vi "Result View.vi"(9 "TestCase map":map{string, map{string, path}}(c390), 10 "Test Tree":refnum<class "Test Tree.lvclass">) -> ()   [LabVIEW 2020]
uses:
  Helper Classes/Test Tree/Test Tree.lvclass
  Helper Classes/Test Tree/Test Tree.lvclass/Test Tree.ctl
panel:
  in  "Test Results":string[](tree)
  in  "Filter fails":bool
  out "Description":string
  out "error out":errorcluster
  in  "error in (no error)":errorcluster
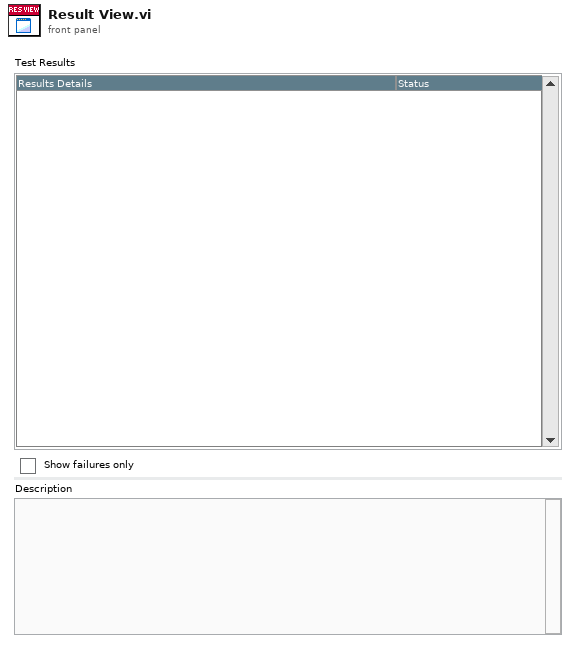
[diagram p1: front panel]
types:
  T1 = cluster{"Message":string, "Message Data":variant}
  T2 = enum32{"Invalid", "Standard", "Closed", "Hidden", "Minimized", "Maximized"}
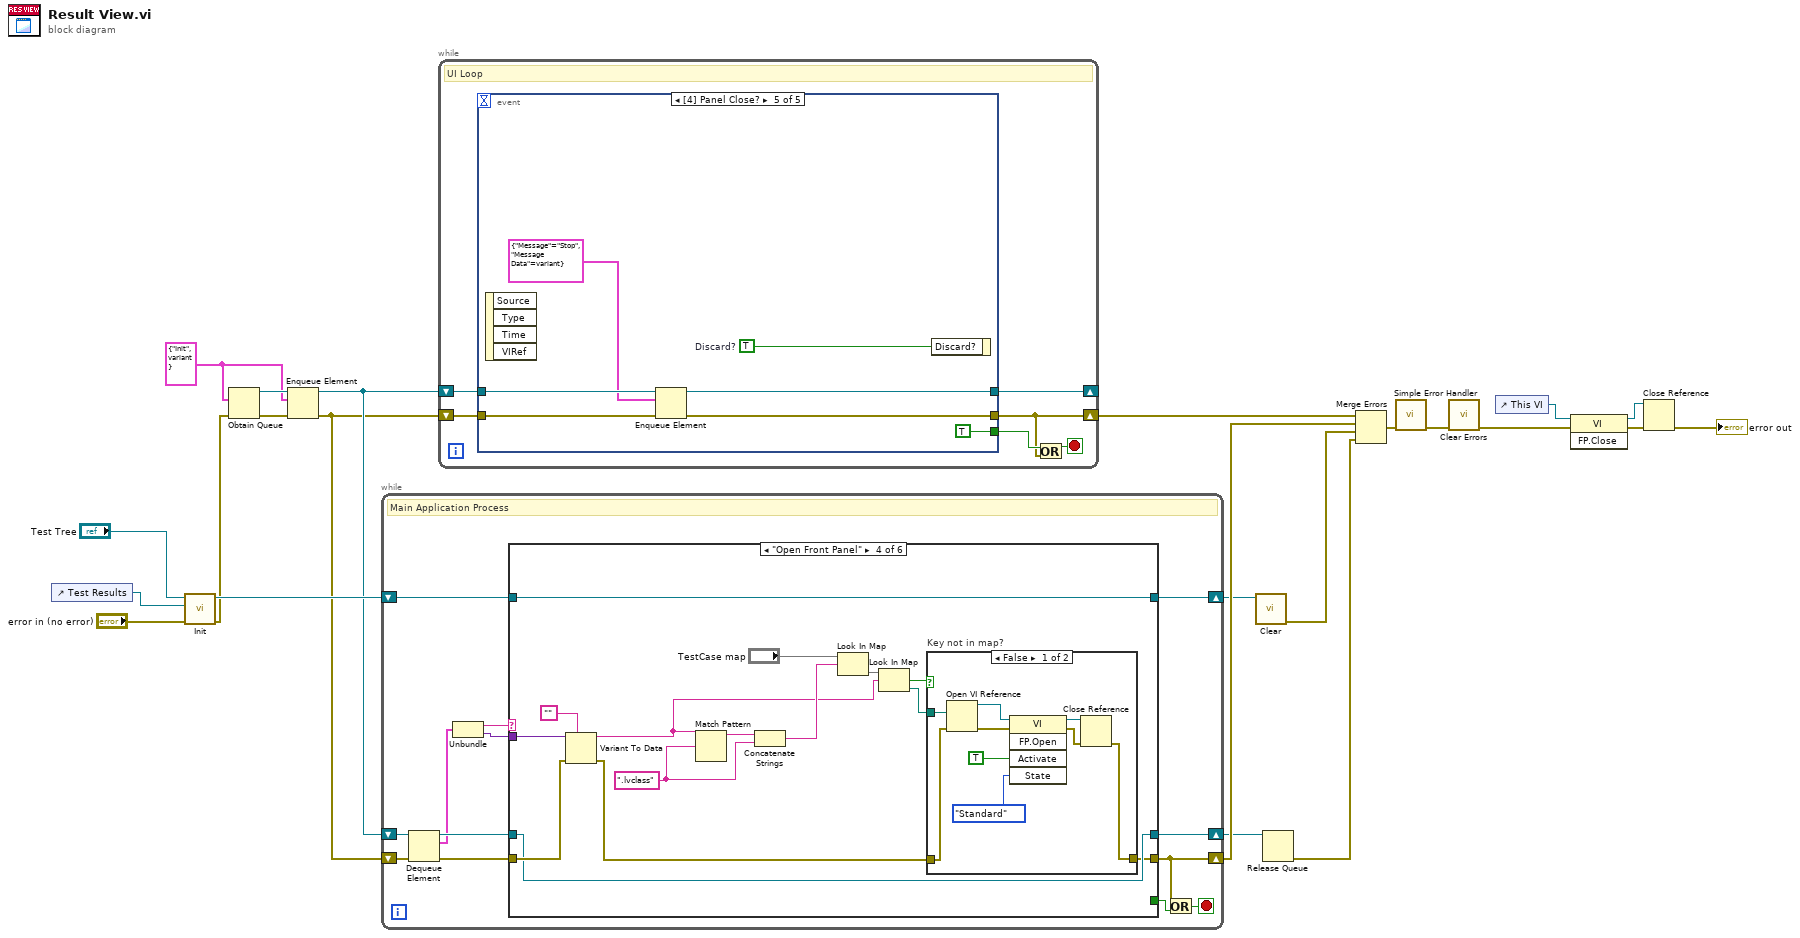
[diagram p0: block diagram]
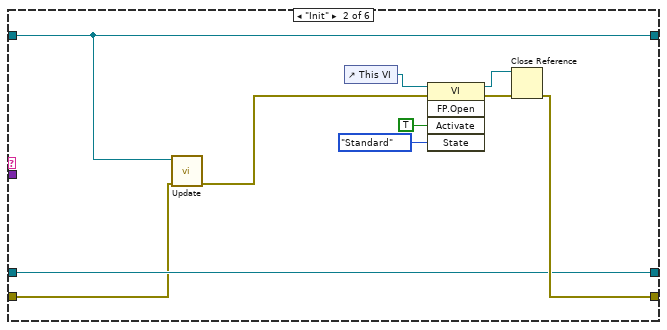
[diagram p3: hidden frame]
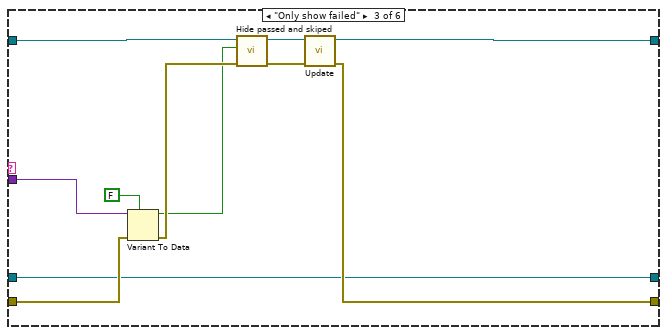
[diagram p4: hidden frame]
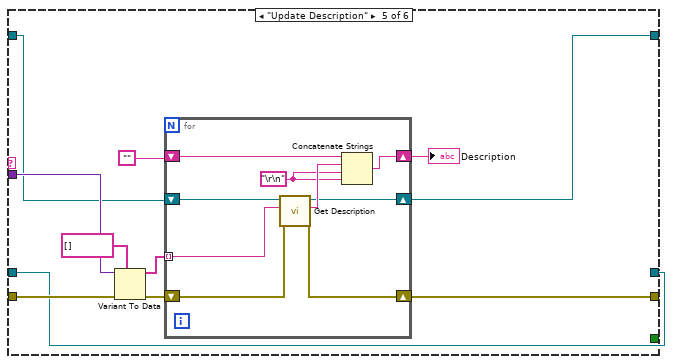
[diagram p6: hidden frame]
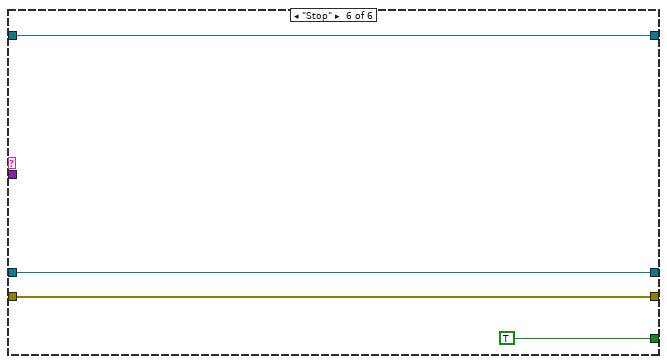
[diagram p7: hidden frame]
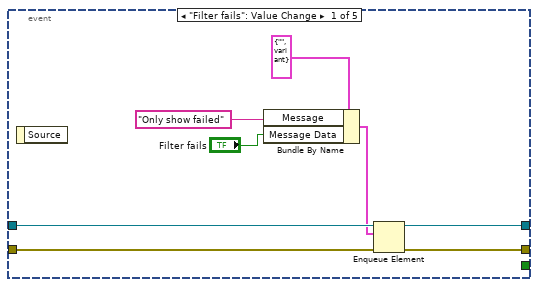
[diagram p8: hidden frame]
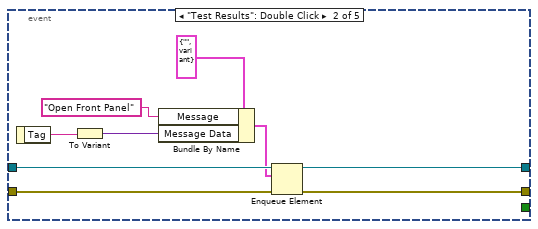
[diagram p9: hidden frame]
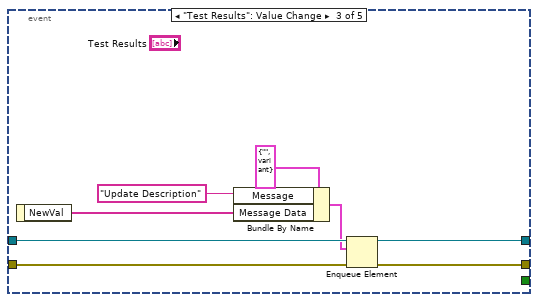
[diagram p10: hidden frame]
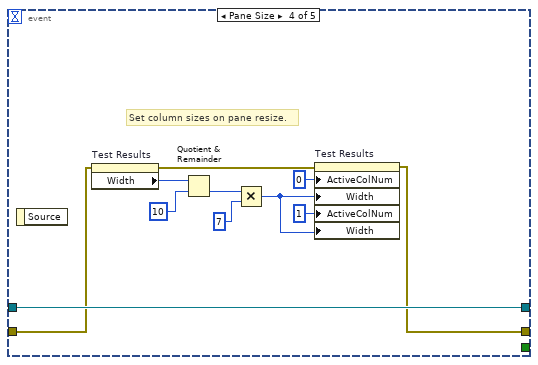
[diagram p11: hidden frame]
diagram:
  w1 = T1 {"Message"="Init", "Message Data"=variant} ("element")
  n1 = control-ref of="Test Results"() -> (w20:refnum<vi>)
  n2 = call-dynamic "Init.vi"("error in (no error)"="error in (no error)", "Test Tree reference"=w20, "Test Tree In"="Test Tree") -> ("error out"=w15:errorcluster, "Test Tree Out"=w16:refnum<class "Test Tree.lvclass">)  [unwired: 7 in]
  n3 = Obtain Queue(element data type=w1, error in (no error)=w15) -> (queue out=w17:refnum<queue>, error out=w13:errorcluster)  [unwired: 3 in, 1 out]
  n4 = Enqueue Element(queue=w17, element=w1, error in (no error)=w13) -> (queue out=w14:refnum<queue>, error out=w12:errorcluster)  [unwired: 1 in, 1 out]
  n5 = while {
    shift-right: [w24] -> w23
    shift-left: w12 -> [w35]
    shift-right: [w31] -> w7
    shift-left: w14 -> [w36]
    shift-right: [w26] -> w8
    shift-left: w16 -> [w27]
    stop <- w25 stop-if-true
    # "Main Application Process"
    n6 = Dequeue Element(queue=w36, error in (no error)=w35) -> (queue out=w34:refnum<queue>, element=w30:T1, error out=w33:errorcluster)  [unwired: 1 in, 1 out]
    n7 = Unbundle(w30) -> ("Message"=w29:string, "Message Data"=w28:variant)
    n8 = case shown="\"Open Front Panel\"" w29 {
      tunnel: w34 -> [w38 w43 w52 w72 w88 w106]
      tunnel: [w38 w43 w52 w72 w88 w106] -> w31
      tunnel: w33 -> [w39 w41 w60 w75 w96 w107]
      tunnel: [w39 w44 w54 w71 w91 w107] -> w24
      tunnel: [_ _ _ _ _ TRUE] -> w32
      tunnel: w28 -> [_ _ w59 w74 w95 _]
      tunnel: w27 -> [w37 w40 w51 w70 w86 w109]
      tunnel: [w37 w40 w50 w70 w87 w109] -> w26
      frame Default {
      }
      frame "Init" {
        n9 = call "Update.vi"("error in (no error)"=w41, "Test Tree In"=w40) -> ("error out"=w42:errorcluster)  [unwired: 8 in, 1 out]
        n10 = control-ref of="This VI"() -> (w47:refnum<vi>)
        n11 = invoke on="Invoke Node" class="VI" method="FP.Open"(reference=w47, error in=w42, "Activate"=TRUE ("Activate?"), "State"=T2."Standard") -> (reference out=w45:refnum<vi>, error out=w46:errorcluster)  [unwired: 1 in, 3 out]
        n12 = Close Reference(reference=w45, error in (no error)=w46) -> (error out=w44:errorcluster)
      }
      frame "Only show failed" {
        n13 = Variant To Data(error in=w60, type=FALSE, Variant=w59) -> (data=w53:bool, error out=w56:errorcluster)
        n14 = call "Hide passed and skiped.vi"("error in (no error)"=w56, "Hide passed/skiped?"=w53, "Test Tree In"=w51) -> ("error out"=w55:errorcluster, "Test Tree Out"=w57:refnum<class "Test Tree.lvclass">)  [unwired: 7 in]
        n15 = call "Update.vi"("error in (no error)"=w55, "Test Tree In"=w57) -> ("error out"=w54:errorcluster, "Test Tree Out"=w50:refnum<class "Test Tree.lvclass">)  [unwired: 8 in]
      }
      frame "Open Front Panel" {
        w64 = ".lvclass" ("regular expression")
        n16 = Variant To Data(error in=w75, type="" ("Empty String Constant"), Variant=w74) -> (data=w63:string, error out=w62:errorcluster)
        n17 = Match Pattern(string=w63, regular expression=w64) -> (before substring=w65:string)  [unwired: 1 in, 3 out]
        n18 = Concatenate Strings(w65, w64) -> (w68:string)
        n19 = Look In Map(map="TestCase map", key=w68) -> (value=w66:map{string, path})  [unwired: 1 in, 1 out]
        n20 = Look In Map(map=w66, key=w63) -> (key not found?=w61:bool, value=w67:path)  [unwired: 1 in]
        n21 = case "Key not in map?" shown="False" w61 {
          tunnel: [w80 w85] -> w71
          tunnel: w67 -> [w79 _]
          tunnel: w62 -> [w76 w85]
          frame False {
            n22 = Open VI Reference(vi path=w79, error in (no error)=w76) -> (vi reference=w78:refnum<vi>, error out=w77:errorcluster)  [unwired: 4 in]
            n23 = invoke class="VI" method="FP.Open"(reference=w78, error in=w77, "Activate"=TRUE ("Activate?"), "State"=T2."Standard") -> (reference out=w81:refnum<vi>, error out=w82:errorcluster)  [unwired: 1 in, 3 out]
            n24 = Close Reference(reference=w81, error in (no error)=w82) -> (error out=w80:errorcluster)
          }
          frame True {
          }
        }
      }
      frame "Update Description" {
        n25 = Variant To Data(error in=w96, type=string[] [], Variant=w95) -> (data=w93:string[], error out=w92:errorcluster)
        n26 = for {
          tunnel: w93 -> [w105] mode=indexing
          shift-right: [w103] -> w91
          shift-left: w92 -> [w104]
          shift-right: [w102] -> w89
          shift-left: "" ("Empty String Constant") -> [w101]
          shift-right: [w97] -> w87
          shift-left: w86 -> [w98]
          w99 = "\r\n" ("End of Line Constant")
          n27 = call "Get Description.vi"("error in (no error)"=w104, "Tag"=w105, "Test Tree In"=w98) -> ("error out"=w103:errorcluster, "Description"=w100:string, "Test Tree Out"=w97:refnum<class "Test Tree.lvclass">)  [unwired: 5 in, 1 out]
          n28 = Concatenate Strings(w101, w100, w99, w99) -> (w102:string)
        }
        "Description" <- w89
      }
      frame "Stop" {
      }
    }
    n29 = Or(x=w24, y=w32) -> (x .or. y?=w25:bool)
  }
  n30 = while {
    shift-right: [w110] -> w22
    shift-left: w12 -> [w114]
    shift-right: [w112] -> _
    shift-left: w14 -> [w115]
    stop <- w111 stop-if-true
    # "UI Loop"
    n31 = event shown="[4] Panel Close?" {
      selector: _ -> [_ _ _ _ _]
      dyn-events: _ -> [_ _ _ _ _]
      timeout: _ -> [_ _ _ _ _]
      tunnel: w115 -> [w123 w132 w140 w151 w157]
      tunnel: w114 -> [w121 w131 w139 w141 w154]
      tunnel: [w120 w129 w138 w142 w155] -> w110
      tunnel: [w122 w130 w137 w151 w156] -> w112
      tunnel: [_ _ _ _ TRUE] -> w113
      event "Filter fails": Value Change {
        n32 = event-data() -> ()  [unwired: 1 in, 1 out]
        n33 = Bundle By Name(cluster=T1 {"Message"="", "Message Data"=variant} ("element"), "Message"="Only show failed", "Message Data"="Filter fails") -> (w118:T1)
        n34 = Enqueue Element(queue=w123, element=w118, error in (no error)=w121) -> (queue out=w122:refnum<queue>, error out=w120:errorcluster)  [unwired: 1 in, 1 out]
      }
      event "Test Results": Double Click {
        n35 = event-data() -> ("Tag"=w128:string)  [unwired: 1 in]
        n36 = To Variant(anything=w128) -> (Variant=w125:variant)
        n37 = Bundle By Name(cluster=T1 {"Message"="", "Message Data"=variant} ("element"), "Message"="Open Front Panel", "Message Data"=w125) -> (w126:T1)
        n38 = Enqueue Element(queue=w132, element=w126, error in (no error)=w131) -> (queue out=w130:refnum<queue>, error out=w129:errorcluster)  [unwired: 1 in, 1 out]
      }
      event "Test Results": Value Change {
        n39 = event-data() -> ("NewVal"=w133:string[])  [unwired: 1 in]
        n40 = Bundle By Name(cluster=T1 {"Message"="", "Message Data"=variant} ("element"), "Message"="Update Description", "Message Data"=w133) -> (w135:T1)
        n41 = Enqueue Element(queue=w140, element=w135, error in (no error)=w139) -> (queue out=w137:refnum<queue>, error out=w138:errorcluster)  [unwired: 1 in, 1 out]
      }
      event Pane Size {
        # "Set column sizes on pane resize."
        n42 = event-data() -> ()  [unwired: 1 in, 1 out]
        n43 = property on="Test Results" class="Tree (strict)"(error in=w141) -> (error out=w143:errorcluster, "Width"=w144:u32)  [unwired: 1 in, 1 out]
        n44 = Quotient & Remainder(x=w144, y=u32 10) -> (floor(x/y)=w148:u32)  [unwired: 1 out]
        n45 = Multiply(x=w148, y=u32 7) -> (x*y=w145:u32)
        n46 = property on="Test Results" class="Tree (strict)"(error in=w143, "ActiveColNum"=0 ("Active Cell:Active Column Number"), "Width"=w145, "ActiveColNum"=1 ("Active Cell:Active Column Number"), "Width"=w145) -> (error out=w142:errorcluster)  [unwired: 1 in, 1 out]
      }
      event Panel Close? {
        w158 = TRUE  # Discard?
        n47 = event-data() -> ()  [unwired: 1 in, 4 out]
        n48 = Enqueue Element(queue=w157, element=T1 {"Message"="Stop", "Message Data"=variant}, error in (no error)=w154) -> (queue out=w156:refnum<queue>, error out=w155:errorcluster)  [unwired: 1 in, 1 out]
        n49 = event-data ("Event Filter Node")("Discard?"=w158) -> ()  [unwired: 1 in, 1 out]
      }
    }
    n50 = Or(x=w113, y=w110) -> (x .or. y?=w111:bool)
  }
  n51 = call-dynamic "Clear.vi"("Test Tree In"=w8) -> ("error out"=w6:errorcluster)  [unwired: 9 in, 1 out]
  n52 = Release Queue(queue=w7) -> (error out=w5:errorcluster)  [unwired: 2 in, 2 out]
  n53 = Merge Errors(w22, w23, w6, w5) -> (w21:errorcluster)
  n54 = call <vilib>:"Simple Error Handler.vi"("error in (no error)"=w21) -> ("error out"=w4:errorcluster)  [unwired: 4 in, 4 out]
  n55 = call <vilib>:"Clear Errors.vi"("error in (no error)"=w4) -> ("error out"=w3:errorcluster)  [unwired: 5 in, 1 out]
  n56 = control-ref of="This VI"() -> (w9:refnum<vi>)
  n57 = invoke on="Invoke Node" class="VI" method="FP.Close"(reference=w9, error in=w3) -> (reference out=w11:refnum<vi>, error out=w10:errorcluster)  [unwired: 1 in, 1 out]
  n58 = Close Reference(reference=w11, error in (no error)=w10) -> (error out=→"error out":errorcluster)
